vi "Load View to SubPanel.vi"(8 "error in (no error)":errorcluster, 10 "SubPnl Refnum":refnum<vi>, 11 "UI View in":refnum<class "UI View.lvclass">) -> (0 "error out":errorcluster, 3 "UI View out":refnum<class "UI View.lvclass">)   [LabVIEW 2013, in "SET Project Editor.lvlib" / "UI View.lvclass"]
uses:
  UI View.lvclass
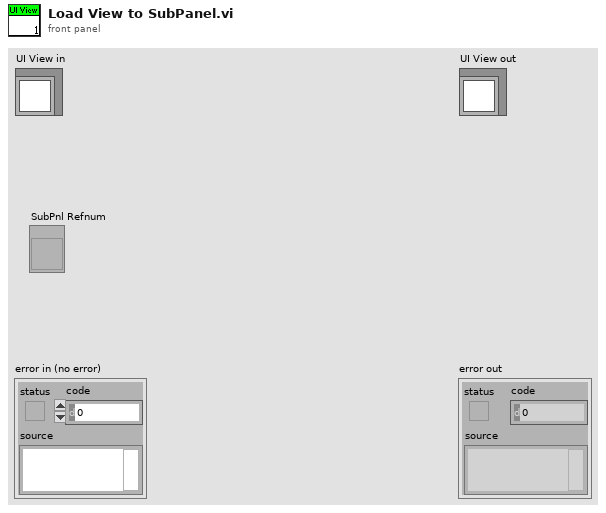
[diagram p1: front panel]
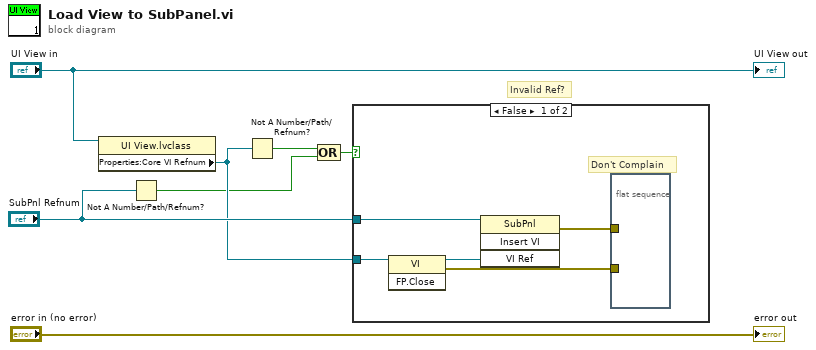
[diagram p0: block diagram]
diagram:
  # "Invalid Ref?"
  n1 = property class="UI View.lvclass"(reference="UI View in") -> ("Properties:Core VI Refnum"=w6:refnum<vi>)  [unwired: 1 in, 2 out]
  n2 = Not A Number/Path/Refnum?(number/path/refnum="SubPnl Refnum") -> (NaN/Path/Refnum?=w4:bool)
  n3 = Not A Number/Path/Refnum?(number/path/refnum=w6) -> (NaN/Path/Refnum?=w5:bool)
  n4 = Compound Arithmetic op=OR(w5, w4) -> (w3:bool)
  n5 = case shown="False" w3 {
    tunnel: "SubPnl Refnum" -> [w11 _]
    tunnel: w6 -> [w10 _]
    frame False {
      # "Don't Complain"
      n6 = invoke class="VI" method="FP.Close"(reference=w10) -> (reference out=w12:refnum<vi>, error out=w8:errorcluster)  [unwired: 2 in, 1 out]
      n7 = invoke class="SubPnl" method="Insert VI"(reference=w11, "VI Ref"=w12) -> (error out=w9:errorcluster)  [unwired: 2 in, 3 out]
      n8 = flat-sequence {
        tunnel: w9 -> [_]
        tunnel: w8 -> [_]
        frame #0 {
        }
      }
    }
    frame True {
    }
  }
  "error out" <- "error in (no error)"
  "UI View out" <- "UI View in"
